vi "test.vi"() -> ()   [LabVIEW 2019]
uses:
  <userlib>/gfitsio/cfitsio-bitpix.ctl
  <userlib>/gfitsio/gfitsio-write-image-subset-i32-2d.vi
  <userlib>/gfitsio/gfitsio-read-image-subset-i32-2d.vi
  <vilib>/picture/picture.llb/Draw True-Color Pixmap.vi
  <userlib>/gfitsio/gfitsio.lvlib
panel:
  out "header":string[](array[string])
  in  "Tab Control":enum32{"Complete Image", "Red", "Green", "Blue"}(tab)
  out "Complete Image":picture
  out "Red":picture
  out "Green":picture
  out "Blue":picture
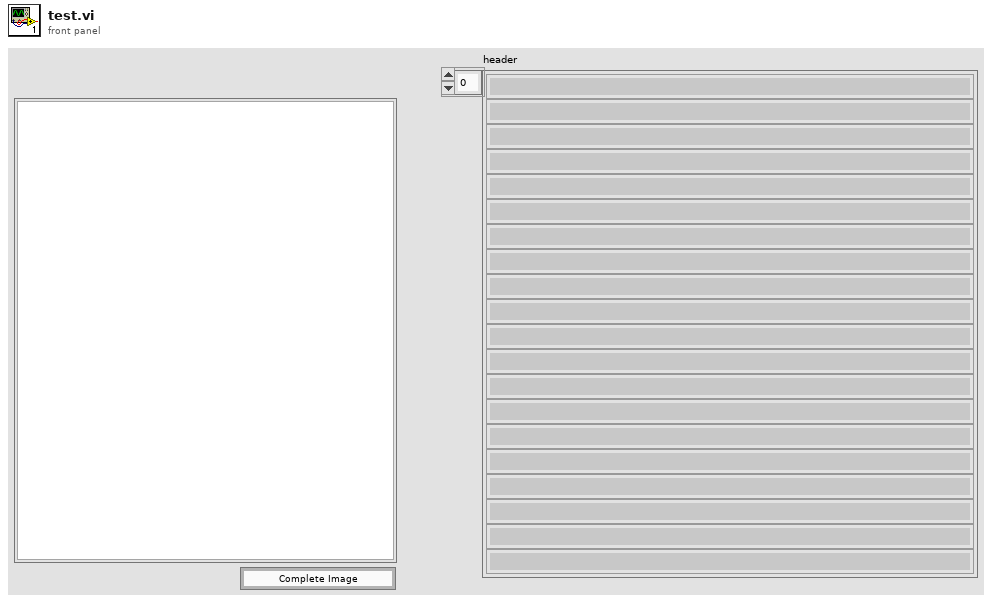
[diagram p1: front panel]
types:
  T1 = enum16{"open", "open or create", "create", "create or replace"}
  T2 = enum16{"open", "open or create", "create or replace", "create", "open (read only)"}
  T3 = typedef "gfitsio.lvlib/cfitsio-bitpix.ctl" = i32
  T4 = typedef "gfitsio.lvlib/gfitsio-refnum.ctl" = refnum<k1>
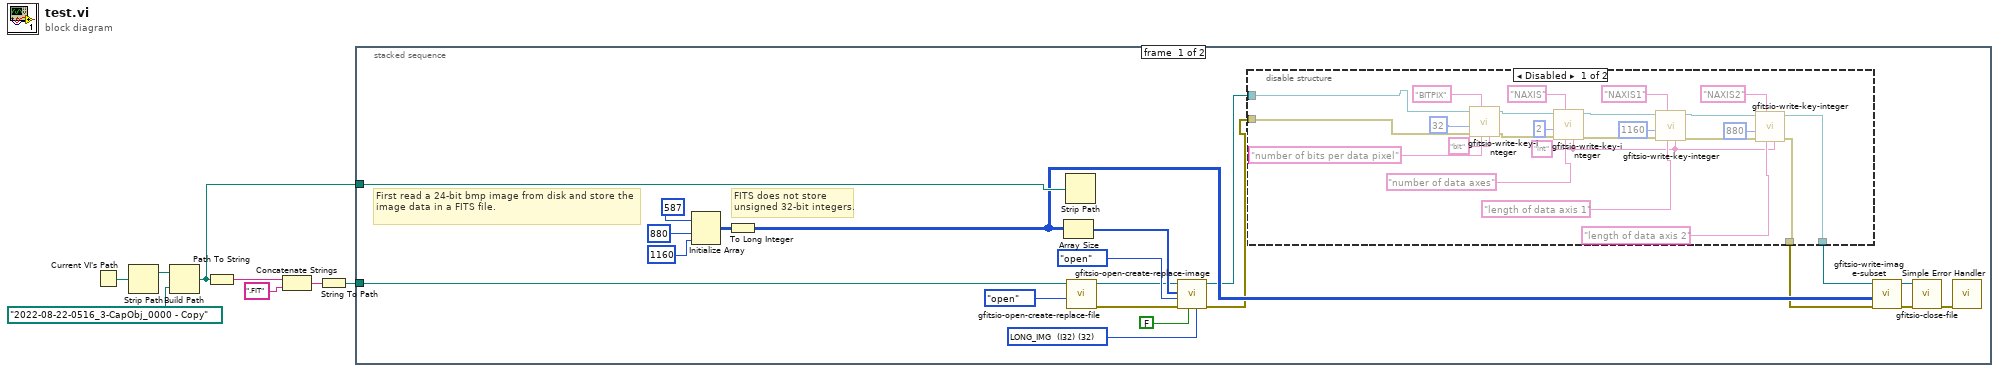
[diagram p0: block diagram]
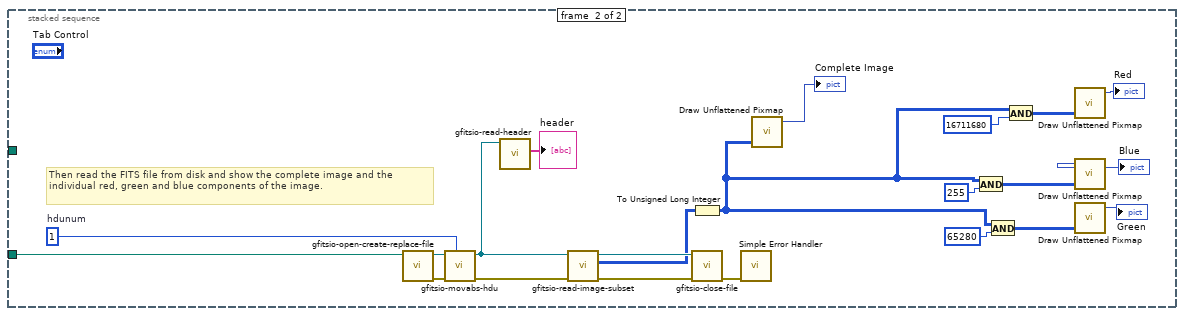
[diagram p3: hidden frame]
diagram:
  n1 = Current VI's Path() -> (path=w6:path)
  n2 = Strip Path(path=w6) -> (stripped path=w7:path)  [unwired: 1 out]
  n3 = Build Path(base path=w7, name or relative path=path "2022-08-22-0516_3-CapObj_0000 - Copy" ("path to BMP file")) -> (appended path=w2:path)
  n4 = Path To String(path=w2) -> (string=w3:string)
  n5 = Concatenate Strings(w3, ".FIT" ("string")) -> (w5:string)
  n6 = String To Path(string=w5) -> (path=w1:path)
  n7 = stacked-sequence {
    tunnel: w2 -> [w29 _]
    tunnel: w1 -> [w9 w57]
    frame #0 {
      w22 = T3 32 items=["<invalid type>"=0, "BYTE_IMG  (U8)"=8, "SHORT_IMG  (I16)"=16, "USHORT_IMG  (U16)"=20, "LONG_IMG  (I32)"=32, "ULONG_IMG  (U32)"=40, "FLOAT_IMG  (SGL)"=-32, "DOUBLE_IMG  (DBL)"=-64] ("image data type")
      # "First read a 24-bit bmp image from disk and store the image data in a FITS file."
      # "FITS does not store unsigned 32-bit integers."
      n8 = Initialize Array(u32 587 ("element"), 880 ("dimension size"), 1160 ("dimension size")) -> (w19:u32[][])
      n9 = To Long Integer(number=w19) -> (32bit integer=w24:i32[][])
      n10 = Array Size(array=w24) -> (size(s)=w23:i32[])
      n11 = Strip Path(path=w29) -> ()  [unwired: 2 out]
      n12 = call <userlib>:"gfitsio-open-create-replace-file.vi"("function (open)"=T2."open", "file path (dialog if empty)"=w9) -> ("error out"=w17:errorcluster, "gfits refnum"=w13:T4)  [unwired: 7 in, 1 out]
      n13 = call <userlib>:"gfitsio-open-create-replace-image.vi"("image data type"=w22, "advisory dialog? (display:T)"=FALSE, "error in (no error)"=w17, "function (create or replace)"=T1."open" ("function (open or create)"), "naxes"=w23, "gfits refnum"=w13) -> ("error out"=w10:errorcluster, "dup gfits refnum"=w11:T4)  [unwired: 3 in, 1 out]
      n14 = disable-structure shown="Disabled" {
        disable-tunnel: [w53 w54] -> w16
        disable-tunnel: [w52 w55] -> w12
        disable-tunnel: w11 -> [w31 w55]
        disable-tunnel: w10 -> [w30 w54]
        frame Disabled {
          w32 = "int" ("units")
          n15 = call <userlib>:"gfitsio-write-key-integer.vi"("units"="bit", "comment"="number of bits per data pixel", "keyname"="BITPIX", "error in (no error)"=w30, "value"=32 ("default value"), "gfits refnum"=w31) -> ("error out"=w44:errorcluster, "dup gfits refnum"=w45:T4)  [unwired: 4 in]
          n16 = call <userlib>:"gfitsio-write-key-integer.vi"("units"=w32, "comment"="number of data axes", "keyname"="NAXIS", "error in (no error)"=w44, "value"=2, "gfits refnum"=w45) -> ("error out"=w39:errorcluster, "dup gfits refnum"=w40:T4)  [unwired: 4 in]
          n17 = call <userlib>:"gfitsio-write-key-integer.vi"("units"=w32, "comment"="length of data axis 1", "keyname"="NAXIS1", "error in (no error)"=w39, "value"=1160, "gfits refnum"=w40) -> ("error out"=w35:errorcluster, "dup gfits refnum"=w38:T4)  [unwired: 4 in]
          n18 = call <userlib>:"gfitsio-write-key-integer.vi"("units"=w32, "comment"="length of data axis 2", "keyname"="NAXIS2", "error in (no error)"=w35, "value"=880, "gfits refnum"=w38) -> ("error out"=w53:errorcluster, "dup gfits refnum"=w52:T4)  [unwired: 4 in]
        }
        frame Enabled {
        }
      }
      n19 = call-poly <userlib>:"gfitsio-write-image-subset.vi"("error in (no error)"=w16, "data"=w24, "gfits refnum"=w12) -> ("error out"=w28:errorcluster, "dup gfits refnum"=w27:T4)  [unwired: 7 in]
      n20 = call <userlib>:"gfitsio-close-file.vi"("error in (no error)"=w28, "gfits refnum"=w27) -> ("error out"=w21:errorcluster)  [unwired: 8 in, 1 out]
      n21 = call <vilib>:"Simple Error Handler.vi"("error in (no error)"=w21) -> ()  [unwired: 4 in, 5 out]
    }
    frame #1 {
      w72 = 1  # hdunum
      # "Then read the FITS file from disk and show the complete image and the individual red, green and blue components of the image."
      n22 = call <userlib>:"gfitsio-open-create-replace-file.vi"("file path (dialog if empty)"=w57) -> ("error out"=w77:errorcluster, "gfits refnum"=w56:T4)  [unwired: 8 in, 1 out]
      n23 = call <userlib>:"gfitsio-movabs-hdu.vi"("hdunum"=w72, "error in (no error)"=w77, "gfits refnum"=w56) -> ("error out"=w76:errorcluster, "dup gfits refnum"=w59:T4)  [unwired: 6 in, 1 out]
      n24 = call <userlib>:"gfitsio-read-header.vi"("gfits refnum"=w59) -> ("header"=→"header":string[])  [unwired: 8 in, 2 out]
      n25 = call-poly <userlib>:"gfitsio-read-image-subset.vi"("error in (no error)"=w76, "gfits refnum"=w59) -> ("error out"=w75:errorcluster, "data"=w71:i32[][], "dup gfits refnum"=w74:T4)  [unwired: 7 in]
      n26 = To Unsigned Long Integer(number=w71) -> (unsigned 32bit integer=w60:u32[][])
      n27 = call <userlib>:"gfitsio-close-file.vi"("error in (no error)"=w75, "gfits refnum"=w74) -> ("error out"=w73:errorcluster)  [unwired: 8 in, 1 out]
      n28 = call <vilib>:"Simple Error Handler.vi"("error in (no error)"=w73) -> ()  [unwired: 4 in, 5 out]
      n29 = call-poly <vilib>:"Draw Unflattened Pixmap.vi"("data (RGB format)"=w60) -> ("new picture"=→"Complete Image":picture)  [unwired: 8 in]
      n30 = And(x=w60, y=u32 255) -> (x .and. y?=w67:u32[][])
      n31 = And(x=w60, y=u32 65280) -> (x .and. y?=w64:u32[][])
      n32 = And(x=w60, y=u32 16711680) -> (x .and. y?=w62:u32[][])
      n33 = call-poly <vilib>:"Draw Unflattened Pixmap.vi"("data (RGB format)"=w62) -> ("new picture"=→"Red":picture)  [unwired: 8 in]
      n34 = call-poly <vilib>:"Draw Unflattened Pixmap.vi"("data (RGB format)"=w67) -> ("new picture"=→"Blue":picture)  [unwired: 8 in]
      n35 = call-poly <vilib>:"Draw Unflattened Pixmap.vi"("data (RGB format)"=w64) -> ("new picture"=→"Green":picture)  [unwired: 8 in]
    }
  }
